vi "Connect to Slave.vi"(8 "error in (no error)":errorcluster, 11 "Modbus master in":refnum<class "Modbus Master.lvclass">) -> (0 "error out":errorcluster, 3 "Modbus master out":refnum<class "Modbus Master.lvclass">)   [LabVIEW 2021, in "Modbus Master.lvclass"]
doc: "Initializes a Modbus master instance. If using the <B>Create Modbus Instance</B> VI, this is not necessary. This function will initiate any required bus communication."
uses:
  Modbus Master.lvclass
  D:/my_projects/projects/Algorithms/Labview/21/Modbus_v121c/API/Modbus API.lvclass
  Modbus API.lvclass/Modbus API.ctl
  Read Network Protocol.vi
  Network Protocol/Network Master/Network Master.lvclass
  D:/my_projects/projects/Algorithms/Labview/21/Modbus_v121c/Network Protocol/Network Protocol.lvclass
  Modbus Master.lvclass/Modbus Master.ctl
  Modbus API.lvclass
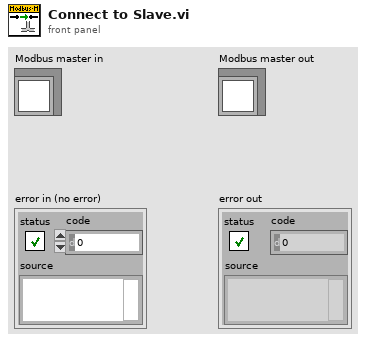
[diagram p1: front panel]
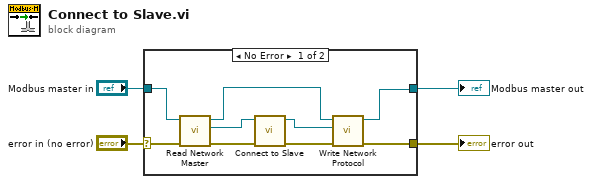
[diagram p0: block diagram]
diagram:
  n1 = case shown="No Error" "error in (no error)" {
    selector: "error in (no error)" -> [w12 w14]
    tunnel: [w9 w15] -> w2
    tunnel: "Modbus master in" -> [w11 w15]
    tunnel: [w10 w14] -> w1
    frame No Error {
      n2 = call "Read Network Master.vi"("error in"=w12, "Modbus master in"=w11) -> ("error out"=w8:errorcluster, "Network Master"=w6:refnum<class "Network Master.lvclass">, "Modbus master out"=w13:refnum<class "Modbus Master.lvclass">)  [unwired: 7 in]
      n3 = call-dynamic "Connect to Slave.vi"("error in (no error)"=w8, "network master in"=w6) -> ("error out"=w7:errorcluster, "network master out"=w5:refnum<class "Network Master.lvclass">)  [unwired: 8 in]
      n4 = call "Write Network Protocol.vi"("error in (no error)"=w7, "Network Protocol"=w5, "Modbus API in"=w13) -> ("error out"=w10:errorcluster, "Modbus API out"=w9:refnum<class "Modbus Master.lvclass">)  [unwired: 7 in]
    }
    frame Error {
    }
  }
  "error out" <- w1
  "Modbus master out" <- w2
